vi "obtainDllPath.vi"() -> (3 "box.dll path":path)   [LabVIEW 2020, in "box.lvlib"]
uses:
  box.lvlib
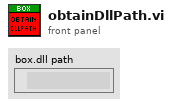
[diagram p1: front panel]
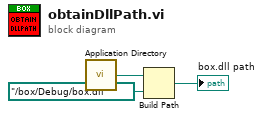
[diagram p0: block diagram]
diagram:
  n1 = call <vilib>:"Application Directory.vi"() -> ("Application Directory"=w3:path)
  n2 = Build Path(base path=w3, name or relative path=path "../box/Debug/box.dll") -> (appended path=→"box.dll path":path)
